vi "GlobalCamSettingsExperiment.vi"() -> ()   [LabVIEW 2019, in "Global.lvlib"]
uses:
  Global.lvlib
  CameraSettings.ctl
panel:
  in  "Camera Settings Exp":T1={"EM Gain :"=150.0, "Pre Amp Gain :"=1.0, "VS Speed [Index] :"=1.0, "VS Amplitude :"=1.0, "Exposure Time [s] :"=0.3, "Temperature :"=0.0, "HS Speed [s]"=0.0, "Gain > 300 :"=FALSE}
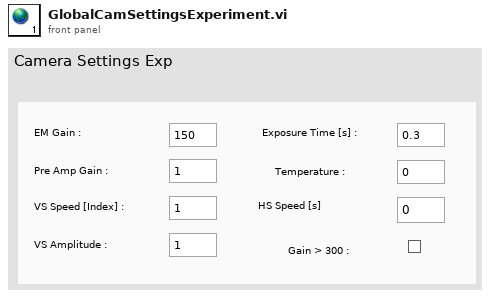
[diagram p1: front panel]
types:
  T1 = typedef "CameraSettings.ctl" = cluster{"EM Gain :":dbl, "Pre Amp Gain :":dbl, "VS Speed [Index] :":dbl, "VS Amplitude :":dbl, "Exposure Time [s] :":dbl, "Temperature :":dbl, "HS Speed [s]":dbl, "Gain > 300 :":bool}
diagram:
